vi "WaitRollTatic.vi"(7 "Game in":refnum<class "Game.lvclass">, 8 "error in (no error)":errorcluster, 9 "first call":bool, 10 "Robot":refnum<class "Robot.lvclass">, 11 "WaitRollTatic in":refnum<class "WaitRollTatic.lvclass">) -> (0 "error out":errorcluster, 2 "Robot out":refnum<class "Robot.lvclass">, 3 "WaitRollTatic out":refnum<class "WaitRollTatic.lvclass">)   [LabVIEW 2023, in "WaitRollTatic.lvclass"]
uses:
  WaitRollTatic.lvclass
  Robot_class/Robot.lvclass
  Game_class/Game.lvclass
  Robot_class/tactics.ctl
  Tactic_class/Tactic.lvclass/Tactic.ctl
  Skillbook_class/Skillbook.lvclass/Skillbook.ctl
  Object_class/Object.lvclass/Object.ctl
  Robot_class/Robot.lvclass/Robot.ctl
  <vilib>/Analysis/_algsub.llb/Real Vector Norm.vi
  Skillbook_class/Read PositionToReceiveRollSkill.vi
  Object_class/Read x.vi
  Object_class/Read y.vi
  Robot_class/Read orientation.vi
  Robot_class/Read dest_x.vi
  Robot_class/Read dest_y.vi
  Robot_class/Read dest_orientation.vi
  Skillbook_class/Read HaltSkill.vi
  Tactic_class/Read Skillbook.vi
  Robot_class/Write tactic.vi
  Skillbook_class/Skillbook.lvclass
  PositionToReceiveRollSkill_class/PositionToReceiveRollSkill.lvclass
  HaltSkill_class/HaltSkill.lvclass
  <vilib>/Analysis/NI_AALPro.lvlib
panel:
  out "Sucsses":bool
  out "x .or. y?":bool
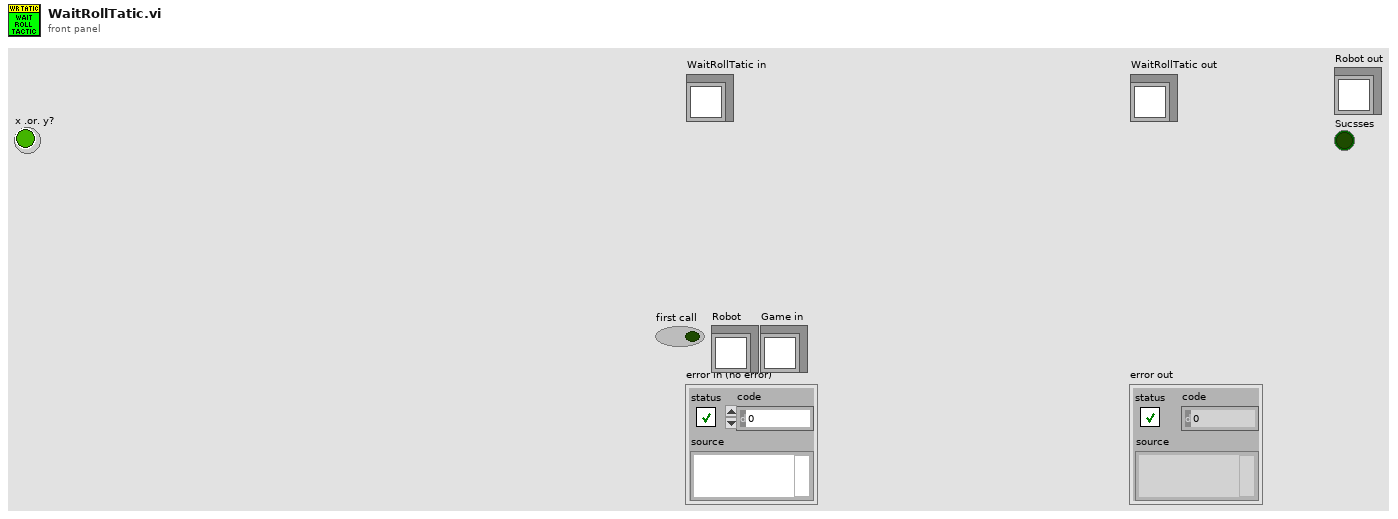
[diagram p1: front panel]
types:
  T1 = typedef "tactics.ctl" = enum16{"ReceivePassInFuturePoint", "Roller", "PrepareRollToPassRollerGoTo", "PrepareRollToPassReceiverGoTo", "WaitRoll", "PositionToRoll", "PenaltyAttacker", "PassObserver", "PenaltyDefense", "TableReceiverTactic", "Test", "DefendGoal", "Marker", "FollowAttacker", "DefendArea", "Shoot", "AttackerAimGoal", "AttackerBallOutOfField", "AttackerBlock", "AttackerStop", "Duelist", "Halt", "ZigZag", "GoTo", "Timeout", "KickToPassReceiver", "PositionToReceivePass", "DefendAreaVSS", "DefendGoalVSS", "KickVSS", "AttackVSS", "DispBallVSS", "PenaltyAttackVSS", "WaitPass"}
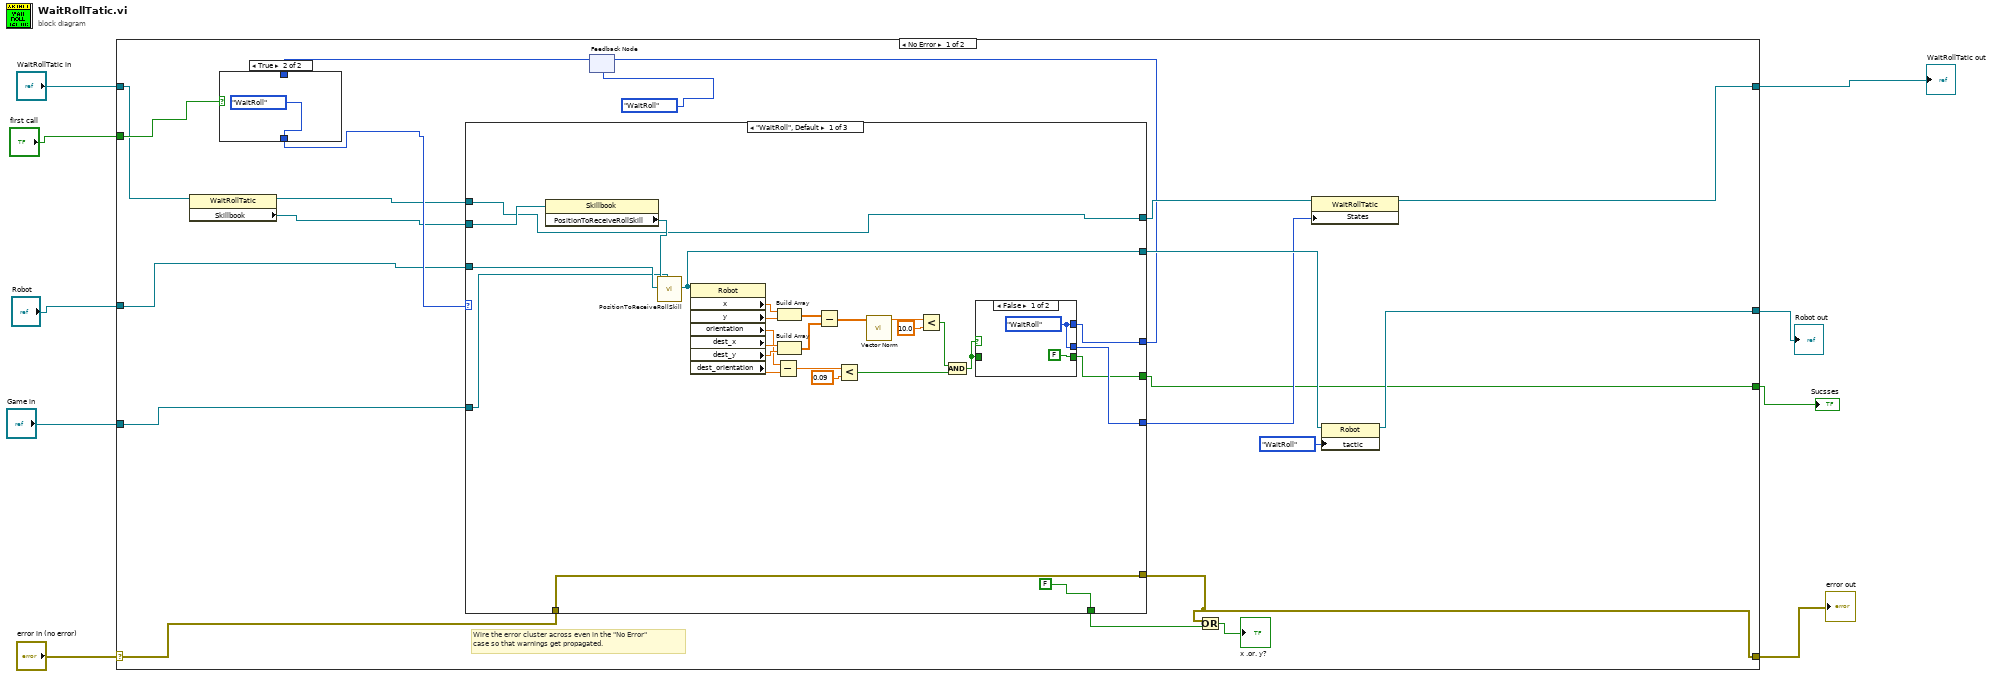
[diagram p0: block diagram]
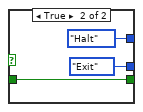
[diagram p2: hidden frame]
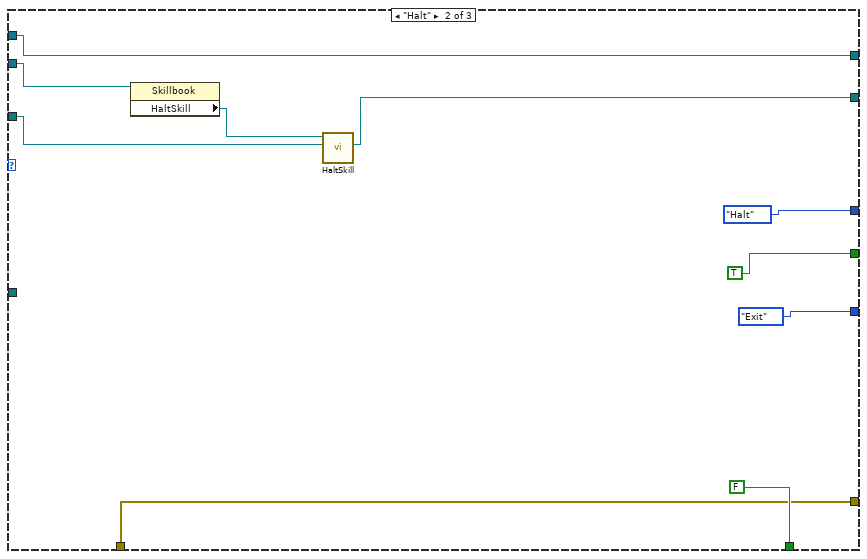
[diagram p3: hidden frame]
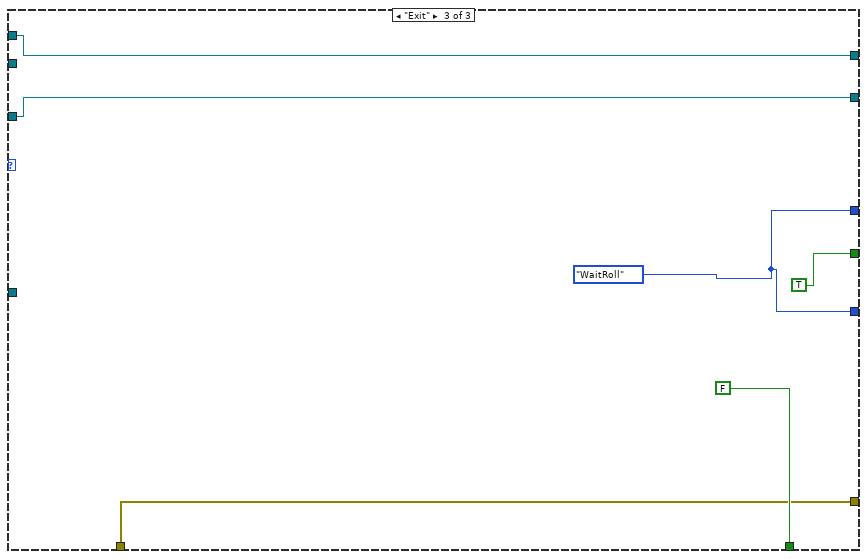
[diagram p4: hidden frame]
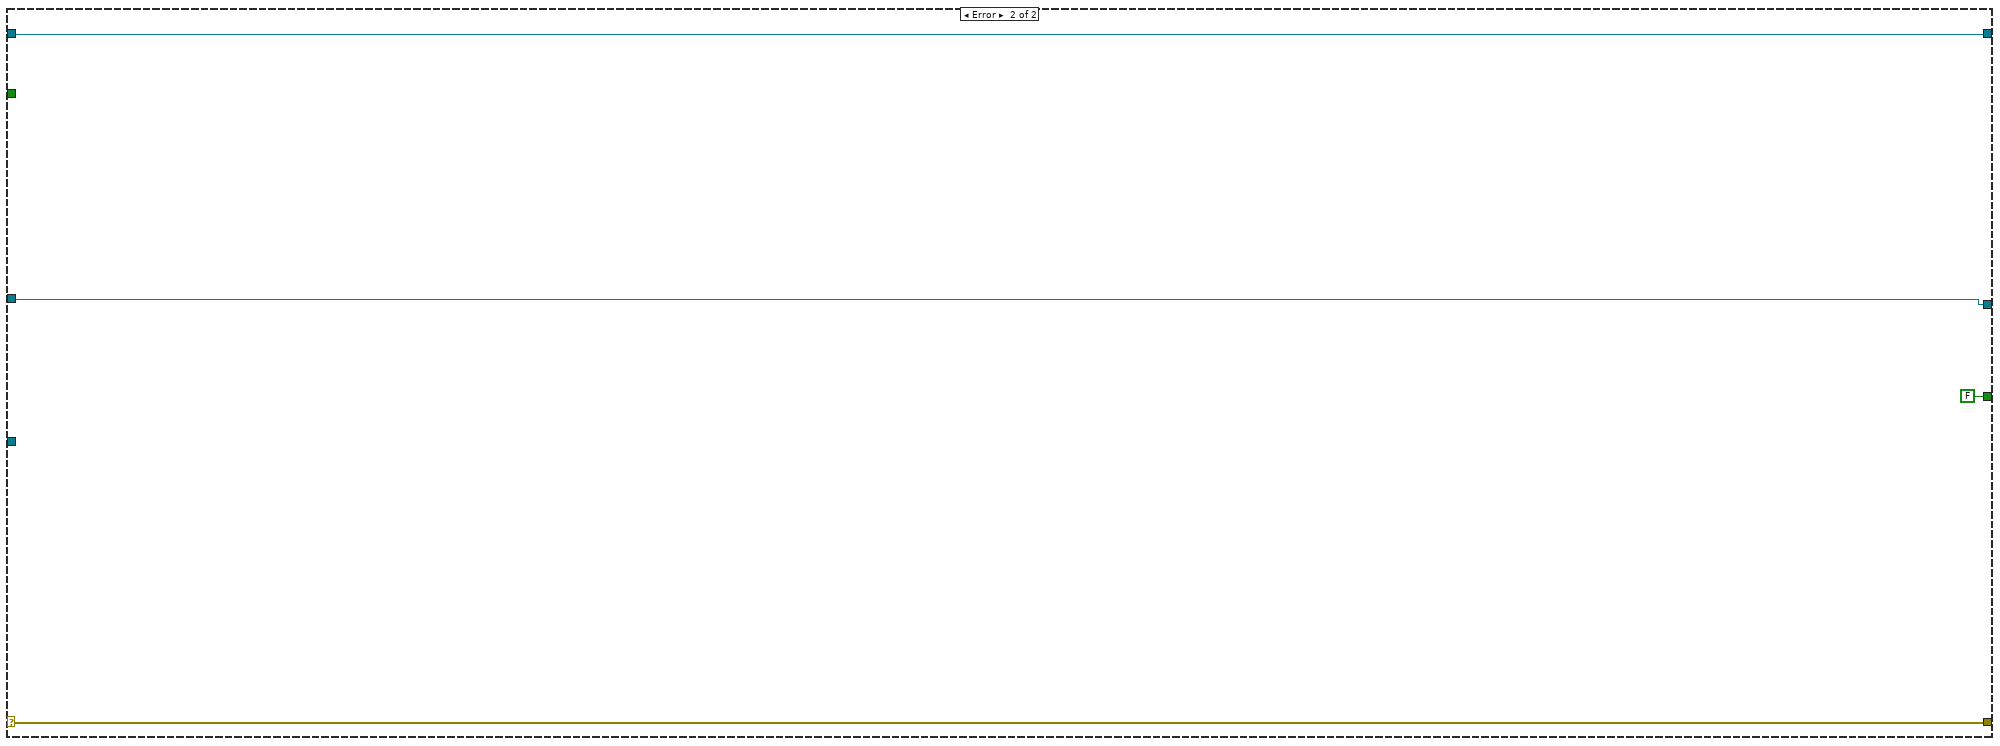
[diagram p6: hidden frame]
diagram:
  n1 = case shown="No Error" "error in (no error)" {
    selector: "error in (no error)" -> [w17 w84]
    tunnel: [w16 w84] -> w8
    tunnel: [w24 w83] -> w6
    tunnel: "WaitRollTatic in" -> [w26 w83]
    tunnel: "first call" -> [w27 _]
    tunnel: "Robot" -> [w19 w81]
    tunnel: "Game in" -> [w18 _]
    tunnel: [w25 w81] -> w2
    tunnel: [w10 FALSE ("x .or. y?")] -> w1
    frame No Error {
      # "Wire the error cluster across even in the \"No Error\"\ncase so that warnings get propagated."
      n2 = property class="WaitRollTatic"(reference=w26) -> (reference out=w21:refnum<class "WaitRollTatic.lvclass">, "Skillbook"=w22:refnum<class "Skillbook.lvclass">)  [unwired: 1 in, 1 out]
      n3 = feedback #1(enum16{"WaitRoll", "Halt", "Exit"}."WaitRoll" ("States")) -> (w30:enum16{"WaitRoll", "Halt", "Exit"})
      n4 = case shown="True" w27 {
        tunnel: [w79 enum16{"WaitRoll", "Halt", "Exit"}."WaitRoll" ("States")] -> w23
        tunnel: w30 -> [w79 _]
        frame False {
        }
        frame True {
        }
      }
      n5 = case shown="\"WaitRoll\", Default" w23 {
        tunnel: w22 -> [w56 w69 _]
        tunnel: w21 -> [w55 w68 w76]
        tunnel: [w55 w68 w76] -> w20
        tunnel: w19 -> [w54 w65 w75]
        tunnel: w18 -> [w53 _ _]
        tunnel: w17 -> [w31 w71 w77]
        tunnel: [w31 w71 w77] -> w16
        tunnel: [FALSE ("x .or. y?") FALSE ("x .or. y?") FALSE ("x .or. y?")] -> w15
        tunnel: [w34 w66 w75] -> w14
        tunnel: [w51 enum16{"WaitRoll", "Halt", "Exit"}."Halt" ("States") w74] -> w13
        tunnel: [w50 enum16{"WaitRoll", "Halt", "Exit"}."Exit" ("States") w74] -> w12
        tunnel: [w33 TRUE ("x .or. y?") TRUE ("x .or. y?")] -> w10
        frame "WaitRoll", Default {
          n6 = property class="Skillbook"(reference=w56) -> ("PositionToReceiveRollSkill"=w57:refnum<class "PositionToReceiveRollSkill.lvclass">)  [unwired: 1 in, 2 out]
          n7 = call "PositionToReceiveRollSkill.vi"("Game in"=w53, "Robot"=w54, "PositionToReceiveRollSkill in"=w57) -> ("Robot out"=w34:refnum<class "Robot.lvclass">)  [unwired: 6 in, 2 out]
          n8 = property class="Robot"(reference=w34) -> ("x"=w49:dbl, "y"=w48:dbl, "orientation"=w43:dbl, "dest_x"=w47:dbl, "dest_y"=w46:dbl, "dest_orientation"=w42:dbl)  [unwired: 1 in, 2 out]
          n9 = Subtract(x=w43, y=w42) -> (x-y=w38:dbl)
          n10 = Build Array(w49, w48) -> (w45:dbl[])
          n11 = Build Array(w47, w46) -> (w44:dbl[])
          n12 = Subtract(x=w45, y=w44) -> (x-y=w41:dbl[])
          n13 = Less?(x=w38, y=0.09) -> (x < y?=w35:bool)
          n14 = call-poly <vilib>:"Vector Norm.vi"("Input Vector"=w41) -> ("norm"=w40:dbl)  [unwired: 9 in, 1 out]
          n15 = Less?(x=w40, y=10.0) -> (x < y?=w36:bool)
          n16 = And(x=w36, y=w35) -> (x .and. y?=w32:bool)
          n17 = case shown="False" w32 {
            tunnel: [w59 enum16{"WaitRoll", "Halt", "Exit"}."Halt" ("States")] -> w51
            tunnel: [w59 enum16{"WaitRoll", "Halt", "Exit"}."Exit" ("States")] -> w50
            tunnel: w32 -> [_ w60]
            tunnel: [FALSE ("x .or. y?") w60] -> w33
            frame False {
              w59 = enum16{"WaitRoll", "Halt", "Exit"}."WaitRoll" ("States")
            }
            frame True {
            }
          }
        }
        frame "Halt" {
          n18 = property class="Skillbook"(reference=w69) -> ("HaltSkill"=w67:refnum<class "HaltSkill.lvclass">)  [unwired: 1 in, 2 out]
          n19 = call-dynamic "HaltSkill.vi"("Robot"=w65, "HaltSkill in"=w67) -> ("Robot out"=w66:refnum<class "Robot.lvclass">)  [unwired: 7 in, 2 out]
        }
        frame "Exit" {
          w74 = enum16{"WaitRoll", "Halt", "Exit"}."WaitRoll" ("States")
        }
      }
      n20 = feedback-in #1(w13) -> ()
      n21 = Or(x=w16, y=w15) -> (x .or. y?=→"x .or. y?":bool)
      n22 = property class="WaitRollTatic"(reference=w20, "States"=w12) -> (reference out=w24:refnum<class "WaitRollTatic.lvclass">)  [unwired: 1 in, 1 out]
      n23 = property class="Robot"(reference=w14, "tactic"=tactics."WaitRoll") -> (reference out=w25:refnum<class "Robot.lvclass">)  [unwired: 1 in, 1 out]
    }
    frame Error {
    }
  }
  "error out" <- w8
  "WaitRollTatic out" <- w6
  "Robot out" <- w2
  "Sucsses" <- w1
